vi "Dispatch Stop.vi"(8 "error in (no error)":errorcluster) -> (0 "error out":errorcluster)   [LabVIEW 2014, in "AMC.lvlib"]
uses:
  AMC.lvlib
  _SubVIs/Globals.vi
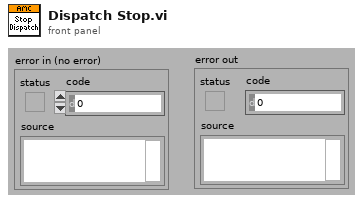
[diagram p1: front panel]
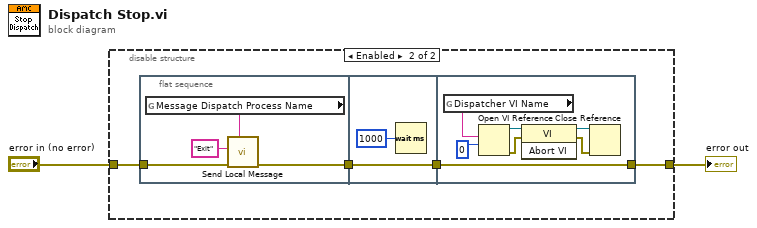
[diagram p0: block diagram]
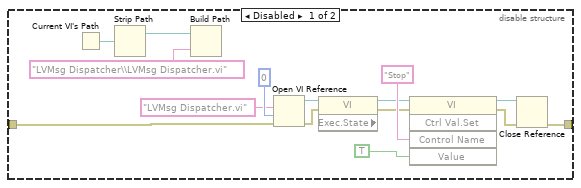
[diagram p2: hidden frame]
diagram:
  n1 = disable-structure shown="Enabled" {
    disable-tunnel: "error in (no error)" -> [w14 w21]
    disable-tunnel: [w13 w18] -> w1
    frame Disabled {
      n2 = Current VI's Path() -> (path=w17:path)
      n3 = Strip Path(path=w17) -> (stripped path=w12:path)  [unwired: 1 out]
      n4 = Build Path(base path=w12, name or relative path="LVMsg Dispatcher\\LVMsg Dispatcher.vi") -> ()  [unwired: 1 out]
      n5 = Open VI Reference(vi path="LVMsg Dispatcher.vi" ("name or relative path"), options=0, error in (no error)=w14) -> (vi reference=w6:refnum<vi>, error out=w5:errorcluster)  [unwired: 3 out]
      n6 = property class="VI" props=["Exec.State"](reference=w6, error in=w5) -> (reference out=w3:refnum<vi>, error out=w4:errorcluster)  [unwired: 1 out]
      n7 = invoke class="VI" method="Ctrl Val.Set"(reference=w3, error in=w4, "Control Name"="Stop", "Value"=TRUE) -> (reference out=w9:refnum<vi>, error out=w8:errorcluster)  [unwired: 1 in, 3 out]
      n8 = Close Reference(reference=w9, error in (no error)=w8) -> (error out=w13:errorcluster)
    }
    frame Enabled {
      n9 = flat-sequence {
        tunnel: w21 -> [w24]
        tunnel: [w22] -> w19
        tunnel: [w27] -> w20
        tunnel: w19 -> [w27]
        tunnel: w20 -> [w30]
        tunnel: [w30] -> w18
        frame #0 {
          n10 = global read "Globals.vi" "Message Dispatch Process Name"() -> (w23:string)
          n11 = call "Send Local Message.vi"("Process (\"\" - local)"=w23, "error in (no error)"=w24, "Message Name"="Exit" ("Name")) -> ("error out"=w22:errorcluster)  [unwired: 4 in, 4 out]
        }
        frame #1 {
          n12 = Wait (ms)(milliseconds to wait=u32 1000) -> ()  [unwired: 1 out]
        }
        frame #2 {
          n13 = global read "Globals.vi" "Dispatcher VI Name"() -> (w28:string)
          n14 = Open VI Reference(vi path=w28, options=0) -> (vi reference=w34:refnum<vi>, error out=w33:errorcluster)  [unwired: 1 in, 3 out]
          n15 = invoke class="VI" method="Abort VI"(reference=w34, error in=w33) -> (reference out=w31:refnum<vi>, error out=w32:errorcluster)  [unwired: 1 in, 1 out]
          n16 = Close Reference(reference=w31, error in (no error)=w32) -> ()  [unwired: 1 out]
        }
      }
    }
  }
  "error out" <- w1
